vi "test_target-steering-values.vi"() -> ()   [LabVIEW 2019]
panel:
  out "error":cluster{"residue":dbl, "residue":dbl}(graph)
  out "intercept":T1(graph)
  in  "대기 시간 (ms)":u32=40
  in  "정지":bool
  out "slope":cluster{"slope":dbl, "slope":dbl}(graph)
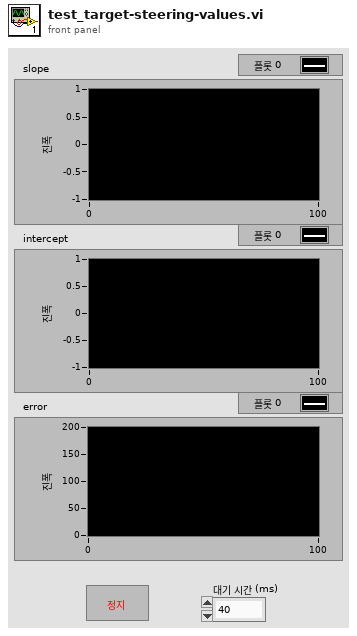
[diagram p1: front panel]
types:
  T1 = cluster{"intercept-l":dbl, "intercept-r":dbl, dbl}
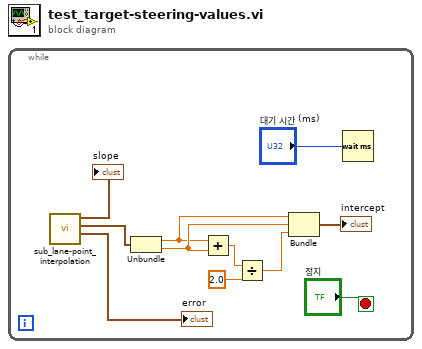
[diagram p0: block diagram]
diagram:
  n1 = while {
    stop <- "정지" stop-if-true
    n2 = call "sub_lane-point_interpolation.vi"() -> ("error"=→"error":cluster{"residue-l":dbl, "residue-r":dbl}, "intercept out"=w7:cluster{"intercept-l":dbl, "intercept-r":dbl}, "slope out"=→"slope":cluster{"slope-l":dbl, "slope-r":dbl})  [unwired: 8 in, 1 out]
    n3 = Unbundle(w7) -> ("intercept-l"=w2:dbl, "intercept-r"=w3:dbl)
    n4 = Add(x=w2, y=w3) -> (x+y=w6:dbl)
    n5 = Divide(x=w6, y=2.0) -> (x/y=w4:dbl)
    n6 = Bundle("intercept-l"=w2, "intercept-r"=w3, w4) -> (→"intercept":T1)  [unwired: 1 in]
    n7 = Wait (ms)(milliseconds to wait="대기 시간 (ms)") -> ()  [unwired: 1 out]
  }
